vi "Parse Trip Association.vi"(1 "Buffer in":string) -> (0 "trip":string)   [LabVIEW 2019, in "PGC2D.lvlib"]
uses:
  PGC2D.lvlib
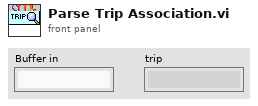
[diagram p1: front panel]
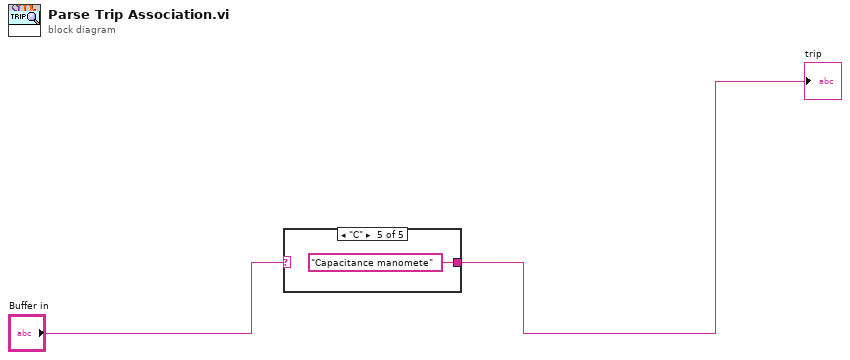
[diagram p0: block diagram]
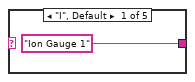
[diagram p2: hidden frame]
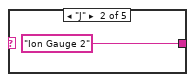
[diagram p3: hidden frame]
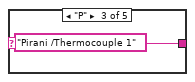
[diagram p4: hidden frame]
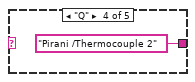
[diagram p5: hidden frame]
diagram:
  n1 = case shown="\"C\"" "Buffer in" {
    tunnel: ["Ion Gauge 1" ("replace string (\"\")") "Ion Gauge 2" ("replace string (\"\")") "Pirani /Thermocouple 1" ("replace string (\"\")") "Pirani /Thermocouple 2" ("replace string (\"\")") "Capacitance manomete" ("replace string (\"\")")] -> w2
    frame "I", Default {
    }
    frame "J" {
    }
    frame "P" {
    }
    frame "Q" {
    }
    frame "C" {
    }
  }
  "trip" <- w2
